vi "test_read-nmea-data2.vi"() -> ()   [LabVIEW 2019] (continued)
,12,307,21,1*5E\n\t\n15:09:51.45\tF9P\t$GPGSV,3,1,09,02,54,318,,04,19,044,,05,36,246,21,06,65,046,22,6*69\n\t\n15:09:51.47\tF9P\t$GPGSV,3,2,09,09,45,075,22,12,24,278,,17,34,153,,19,53,156,,6*63\n\t\n15:09:51.49\tF9P\t$GPGSV,3,3,09,25,12,307,,6*5A\n\t\n15:09:51.51\tF9P\t$GLGSV,2,1,08,69,13,031,,70,73,042,,71,50,204,27,72,03,209,,1*74\n\t\n15:09:51.53\tF9P\t$GLGSV,2,2,08,77,01,327,,84,21,121,08,85,70,063,24,86,35,329,,1*7B\n\t\n15:09:51.55\tF9P\t$GLGSV,2,1,08,69,13,031,,70,73,042,,71,50,204,21,72,03,209,,3*70\n\t\n15:09:51.57\tF9P\t$GLGSV,2,2,08,77,01,327,,84,21,121,12,85,70,063,18,86,35,329,,3*7D\n\t\n15:09:51.59\tF9P\t$GAGSV,2,1,08,02,09,298,,04,66,119,25,09,31,193,36,11,71,357,24,7*7E\n\t\n15:09:51.61\tF9P\t$GAGSV,2,2,08,12,40,102,17,19,27,045,10,25,09,249,,36,25,308,31,7*7E\n\t\n15:09:51.63\tF9P\t$GAGSV,2,1,08,02,09,298,,04,66,119,21,09,31,193,20,11,71,357,20,2*7C\n\t\n15:09:51.65\tF9P\t$GAGSV,2,2,08,12,40,102,,19,27,045,,25,09,249,,36,25,308,,2*7E\n\t\n15:09:51.67\tF9P\t$GBGSV,1,1,03,11,51,130,33,14,86,148,28,33,59,218,26,1*4C\n\t\n15:09:51.69\tF9P\t$GBGSV,1,1,04,08,,,22,11,51,130,25,14,86,148,21,33,59,218,,3*4B\n\t\n15:09:51.71\tF9P\t$GNGLL,3723.58734,N,12656.89105,E,060953.00,A,A*75\n\t\n15:09:51.73\tF9P\t\t\n15:09:51.75\tF9P\t\t\n15:09:51.77\tF9P\t\t\n15:09:51.79\tF9P\t\t\n15:09:51.81\tF9P\t\t\n15:09:51.83\tF9P\t\t\n15:09:51.85\tF9P\t\t\n15:09:51.87\tF9P\t\t\n15:09:51.89\tF9P\t\t\n15:09:51.91\tF9P\t\t\n15:09:51.93\tF9P\t\t\n15:09:51.95\tF9P\t\t\n15:09:51.97\tF9P\t\t\n15:09:51.99\tF9P\t\t\n15:09:52.01\tF9P\t\t\n15:09:52.03\tF9P\t\t\n15:09:52.05\tF9P\t\t\n15:09:52.07\tF9P\t\t\n15:09:52.09\tF9P\t\t\n15:09:52.11\tF9P\t\t\n15:09:52.13\tF9P\t\t\n15:09:52.15\tF9P\t\t\n15:09:52.17\tF9P\t\t\n15:09:52.19\tF9P\t\t\n15:09:52.21\tF9P\t\t\n15:09:52.23\tF9P\t\t\n15:09:52.25\tF9P\t$GNRMC,060954.00,A,3723.58684,N,12656.89052,E,0.440,,250720,,,A,V*1A\n\t\n15:09:52.27\tF9P\t$GNVTG,,T,,M,0.440,N,0.814,K,A*30\n\t\n15:09:52.29\tF9P\t$GNGGA,060954.00,3723.58684,N,12656.89052,E,1,12,0.74,39.4,M,18.5,M,,*7C\n\t\n15:09:52.31\tF9P\t$GNGSA,A,3,12,06,19,05,17,09,02,,,,,,1.38,0.74,1.16,1*0B\n\t\n15:09:52.33\tF9P\t$GNGSA,A,3,85,71,84,,,,,,,,,,1.38,0.74,1.16,2*0A\n\t\n15:09:52.35\tF9P\t$GNGSA,A,3,36,19,11,04,09,12,,,,,,,1.38,0.74,1.16,3*0F\n\t\n15:09:52.37\tF9P\t$GNGSA,A,3,14,11,33,,,,,,,,,,1.38,0.74,1.16,4*0E\n\t\n15:09:52.39\tF9P\t$GPGSV,3,1,09,02,54,318,32,04,19,044,,05,36,246,33,06,65,046,39,1*66\n\t\n15:09:52.41\tF9P\t$GPGSV,3,2,09,09,45,075,33,12,24,278,21,17,34,153,20,19,53,156,34,1*62\n\t\n15:09:52.43\tF9P\t$GPGSV,3,3,09,25,12,307,21,1*5E\n\t\n15:09:52.45\tF9P\t$GPGSV,3,1,09,02,54,318,,04,19,044,,05,36,246,21,06,65,046,29,6*62\n\t\n15:09:52.47\tF9P\t$GPGSV,3,2,09,09,45,075,22,12,24,278,,17,34,153,,19,53,156,,6*63\n\t\n15:09:52.49\tF9P\t$GPGSV,3,3,09,25,12,307,,6*5A\n\t\n15:09:52.51\tF9P\t$GLGSV,2,1,08,69,13,031,,70,73,042,,71,50,204,35,72,03,209,,1*77\n\t\n15:09:52.53\tF9P\t$GLGSV,2,2,08,77,01,327,,84,21,121,07,85,70,063,30,86,35,329,,1*71\n\t\n15:09:52.55\tF9P\t$GLGSV,2,1,08,69,13,031,,70,73,042,,71,50,204,21,72,03,209,,3*70\n\t\n15:09:52.57\tF9P\t$GLGSV,2,2,08,77,01,327,,84,21,121,12,85,70,063,27,86,35,329,,3*71\n\t\n15:09:52.59\tF9P\t$GAGSV,2,1,08,02,09,298,16,04,66,119,40,09,31,193,38,11,71,357,26,7*76\n\t\n15:09:52.61\tF9P\t$GAGSV,2,2,08,12,40,102,28,19,27,045,14,25,09,249,,36,25,308,32,7*75\n\t\n15:09:52.63\tF9P\t$GAGSV,2,1,08,02,09,298,,04,66,119,30,09,31,193,,11,71,357,23,2*7D\n\t\n15:09:52.65\tF9P\t$GAGSV,2,2,08,12,40,102,,19,27,045,,25,09,249,,36,25,308,,2*7E\n\t\n15:09:52.67\tF9P\t$GBGSV,1,1,03,11,50,131,45,14,86,148,37,33,59,218,33,1*47\n\t\n15:09:52.69\tF9P\t$GBGSV,1,1,04,08,,,29,11,50,131,25,14,86,148,,33,59,218,,3*43\n\t\n15:09:52.71\tF9P\t$GNGLL,3723.58684,N,12656.89052,E,060954.00,A,A*7B\n\t\n15:09:52.73\tF9P\t\t\n15:09:52.75\tF9P\t\t\n15:09:52.77\tF9P\t\t\n15:09:52.79\tF9P\t\t\n15:09:52.81\tF9P\t\t\n15:09:52.83\tF9P\t\t\n15:09:52.85\tF9P\t\t\n15:09:52.87\tF9P\t\t\n15:09:52.89\tF9P\t\t\n15:09:52.91\tF9P\t\t\n15:09:52.93\tF9P\t\t\n15:09:52.95\tF9P\t\t\n15:09:52.97\tF9P\t\t\n15:09:52.99\tF9P\t\t\n15:09:53.01\tF9P\t\t\n15:09:53.03\tF9P\t\t\n15:09:53.05\tF9P\t\t\n15:09:53.07\tF9P\t\t\n15:09:53.09\tF9P\t\t\n15:09:53.11\tF9P\t\t\n15:09:53.13\tF9P\t\t\n15:09:53.15\tF9P\t\t\n15:09:53.17\tF9P\t\t\n15:09:53.19\tF9P\t\t\n15:09:53.21\tF9P\t\t\n15:09:53.23\tF9P\t\t\n15:09:53.25\tF9P\t$GNRMC,060955.00,A,3723.58663,N,12656.88996,E,1.556,250.04,250720,,,A,V*08\n\t\n15:09:53.27\tF9P\t$GNVTG,250.04,T,,M,1.556,N,2.883,K,A*26\n\t\n15:09:53.29\tF9P\t$GNGGA,060955.00,3723.58663,N,12656.88996,E,1,12,0.78,38.7,M,18.5,M,,*7A\n\t\n15:09:53.31\tF9P\t$GNGSA,A,3,12,06,19,05,17,09,02,,,,,,1.55,0.78,1.34,1*0C\n\t\n15:09:53.33\tF9P\t$GNGSA,A,3,85,71,84,,,,,,,,,,1.55,0.78,1.34,2*0D\n\t\n15:09:53.35\tF9P\t$GNGSA,A,3,36,19,11,04,09,12,,,,,,,1.55,0.78,1.34,3*08\n\t\n15:09:53.37\tF9P\t$GNGSA,A,3,14,11,33,,,,,,,,,,1.55,0.78,1.34,4*09\n\t\n15:09:53.39\tF9P\t$GPGSV,3,1,09,02,54,318,32,04,19,044,20,05,36,246,36,06,65,046,38,1*60\n\t\n15:09:53.41\tF9P\t$GPGSV,3,2,09,09,45,075,34,12,24,278,21,17,34,153,23,19,53,156,28,1*6B\n\t\n15:09:53.43\tF9P\t$GPGSV,3,3,09,25,12,307,21,1*5E\n\t\n15:09:53.45\tF9P\t$GPGSV,3,1,09,02,54,318,,04,19,044,,05,36,246,21,06,65,046,22,6*69\n\t\n15:09:53.47\tF9P\t$GPGSV,3,2,09,09,45,075,23,12,24,278,,17,34,153,,19,53,156,,6*62\n\t\n15:09:53.49\tF9P\t$GPGSV,3,3,09,25,12,307,,6*5A\n\t\n15:09:53.51\tF9P\t$GLGSV,2,1,08,69,13,031,,70,73,042,,71,50,204,31,72,03,209,,1*73\n\t\n15:09:53.53\tF9P\t$GLGSV,2,2,08,77,01,327,,84,21,121,13,85,70,063,23,86,35,329,,1*76\n\t\n15:09:53.55\tF9P\t$GLGSV,2,1,08,69,13,031,,70,73,042,,71,50,204,29,72,03,209,,3*78\n\t\n15:09:53.57\tF9P\t$GLGSV,2,2,08,77,01,327,,84,21,121,16,85,70,063,21,86,35,329,,3*73\n\t\n15:09:53.59\tF9P\t$GAGSV,2,1,08,02,09,298,17,04,66,119,29,09,31,193,28,11,71,357,29,7*76\n\t\n15:09:53.61\tF9P\t$GAGSV,2,2,08,12,40,102,26,19,27,045,08,25,09,249,,36,25,308,27,7*72\n\t\n15:09:53.63\tF9P\t$GAGSV,2,1,08,02,09,298,,04,66,119,25,09,31,193,,11,71,357,22,2*78\n\t\n15:09:53.65\tF9P\t$GAGSV,2,2,08,12,40,102,,19,27,045,,25,09,249,,36,25,308,,2*7E\n\t\n15:09:53.67\tF9P\t$GBGSV,1,1,03,11,50,131,26,14,87,138,29,33,59,218,28,1*41\n\t\n15:09:53.69\tF9P\t$GBGSV,1,1,04,08,,,30,11,50,131,26,14,87,138,28,33,59,218,,3*44\n\t\n15:09:53.71\tF9P\t$GNGLL,3723.58663,N,12656.88996,E,060955.00,A,A*73\n\t\n15:09:53.73\tF9P\t\t\n15:09:53.75\tF9P\t\t\n15:09:53.77\tF9P\t\t\n15:09:53.79\tF9P\t\t\n15:09:53.81\tF9P\t\t\n15:09:53.83\tF9P\t\t\n15:09:53.85\tF9P\t\t\n15:09:53.87\tF9P\t\t\n15:09:53.89\tF9P\t\t\n15:09:53.91\tF9P\t\t\n15:09:53.93\tF9P\t\t\n15:09:53.95\tF9P\t\t\n15:09:53.97\tF9P\t\t\n15:09:53.99\tF9P\t\t\n15:09:54.01\tF9P\t\t\n15:09:54.03\tF9P\t\t\n15:09:54.05\tF9P\t\t\n15:09:54.07\tF9P\t\t\n15:09:54.09\tF9P\t\t\n15:09:54.11\tF9P\t\t\n15:09:54.13\tF9P\t\t\n15:09:54.15\tF9P\t\t\n15:09:54.17\tF9P\t\t\n15:09:54.19\tF9P\t\t\n15:09:54.21\tF9P\t\t\n15:09:54.23\tF9P\t\t\n15:09:54.25\tF9P\t$GNRMC,060956.00,A,3723.58624,N,12656.88943,E,1.511,240.62,250720,,,A,V*02\n\t\n15:09:54.27\tF9P\t$GNVTG,240.62,T,,M,1.511,N,2.799,K,A*20\n\t\n15:09:54.29\tF9P\t$GNGGA,060956.00,3723.58624,N,12656.88943,E,1,12,0.72,37.8,M,18.5,M,,*78\n\t\n15:09:54.31\tF9P\t$GNGSA,A,3,12,06,19,05,17,09,02,,,,,,1.36,0.72,1.16,1*03\n\t\n15:09:54.33\tF9P\t$GNGSA,A,3,85,71,84,,,,,,,,,,1.36,0.72,1.16,2*02\n\t\n15:09:54.35\tF9P\t$GNGSA,A,3,36,19,11,04,09,12,,,,,,,1.36,0.72,1.16,3*07\n\t\n15:09:54.37\tF9P\t$GNGSA,A,3,14,11,33,,,,,,,,,,1.36,0.72,1.16,4*06\n\t\n15:09:54.39\tF9P\t$GPGSV,3,1,09,02,54,318,28,04,19,044,20,05,36,246,29,06,65,046,38,1*65\n\t\n15:09:54.41\tF9P\t$GPGSV,3,2,09,09,45,075,31,12,24,278,22,17,34,153,22,19,53,156,26,1*62\n\t\n15:09:54.43\tF9P\t$GPGSV,3,3,09,25,12,307,22,1*5D\n\t\n15:09:54.45\tF9P\t$GPGSV,3,1,09,02,54,318,,04,19,044,,05,36,246,22,06,65,046,21,6*69\n\t\n15:09:54.47\tF9P\t$GPGSV,3,2,09,09,45,075,21,12,24,278,,17,34,153,,19,53,156,,6*60\n\t\n15:09:54.49\tF9P\t$GPGSV,3,3,09,25,12,307,,6*5A\n\t\n15:09:54.51\tF9P\t$GLGSV,2,1,08,69,13,031,,70,73,042,,71,50,204,26,72,03,209,,1*75\n\t\n15:09:54.53\tF9P\t$GLGSV,2,2,08,77,01,327,,84,21,121,10,85,70,063,29,86,35,329,,1*7F\n\t\n15:09:54.55\tF9P\t$GLGSV,2,1,08,69,13,031,,70,73,042,,71,50,204,22,72,03,209,,3*73\n\t\n15:09:54.57\tF9P\t$GLGSV,2,2,08,77,01,327,,84,21,121,18,85,70,063,21,86,35,329,,3*7D\n\t\n15:09:54.59\tF9P\t$GAGSV,2,1,08,02,09,298,16,04,66,119,26,09,31,193,27,11,71,357,26,7*78\n\t\n15:09:54.61\tF9P\t$GAGSV,2,2,08,12,40,102,22,19,27,045,13,25,09,249,,36,25,308,25,7*7E\n\t\n15:09:54.63\tF9P\t$GAGSV,2,1,08,02,09,298,,04,66,119,25,09,31,193,,11,71,357,20,2*7A\n\t\n15:09:54.65\tF9P\t$GAGSV,2,2,08,12,40,102,,19,27,045,,25,09,249,,36,25,308,,2*7E\n\t\n15:09:54.67\tF9P\t$GBGSV,2,1,05,11,50,131,27,12,,,21,14,87,138,22,15,,,22,1*77\n\t\n15:09:54.69\tF9P\t$GBGSV,2,2,05,33,59,218,31,1*46\n\t\n15:09:54.71\tF9P\t$GBGSV,1,1,03,11,50,131,25,14,87,138,27,33,59,218,,3*44\n\t\n15:09:54.73\tF9P\t$GNGLL,3723.58624,N,12656.88943,E,060956.00,A,A*7B\n\t\n15:09:54.75\tF9P\t\t\n15:09:54.77\tF9P\t\t\n15:09:54.79\tF9P\t\t\n15:09:54.81\tF9P\t\t\n15:09:54.83\tF9P\t\t\n15:09:54.85\tF9P\t\t\n15:09:54.87\tF9P\t\t\n15:09:54.89\tF9P\t\t\n15:09:54.91\tF9P\t\t\n15:09:54.93\tF9P\t\t\n15:09:54.95\tF9P\t\t\n15:09:54.97\tF9P\t\t\n15:09:54.99\tF9P\t\t\n15:09:55.01\tF9P\t\t\n15:09:55.03\tF9P\t\t\n15:09:55.05\tF9P\t\t\n15:09:55.07\tF9P\t\t\n15:09:55.09\tF9P\t\t\n15:09:55.11\tF9P\t\t\n15:09:55.13\tF9P\t\t\n15:09:55.15\tF9P\t\t\n15:09:55.17\tF9P\t\t\n15:09:55.19\tF9P\t\t\n15:09:55.21\tF9P\t\t\n15:09:55.23\tF9P\t\t\n15:09:55.25\tF9P\t$GNRMC,060957.00,A,3723.58600,N,12656.88891,E,1.206,,250720,,,A,V*16\n\t\n15:09:55.27\tF9P\t$GNVTG,,T,,M,1.206,N,2.234,K,A*3F\n\t\n15:09:55.29\tF9P\t$GNGGA,060957.00,3723.58600,N,12656.88891,E,1,12,0.72,37.6,M,18.5,M,,*7F\n\t\n15:09:55.31\tF9P\t$GNGSA,A,3,12,06,19,05,17,09,02,,,,,,1.36,0.72,1.16,1*03\n\t\n15:09:55.33\tF9P\t$GNGSA,A,3,85,71,84,,,,,,,,,,1.36,0.72,1.16,2*02\n\t\n15:09:55.35\tF9P\t$GNGSA,A,3,36,19,11,04,09,12,,,,,,,1.36,0.72,1.16,3*07\n\t\n15:09:55.37\tF9P\t$GNGSA,A,3,14,11,33,,,,,,,,,,1.36,0.72,1.16,4*06\n\t\n15:09:55.39\tF9P\t$GPGSV,3,1,09,02,54,318,27,04,19,044,19,05,36,246,29,06,65,046,32,1*6A\n\t\n15:09:55.41\tF9P\t$GPGSV,3,2,09,09,45,075,30,12,24,278,21,17,34,153,21,19,53,156,25,1*60\n\t\n15:09:55.43\tF9P\t$GPGSV,3,3,09,25,12,307,20,1*5F\n\t\n15:09:55.45\tF9P\t$GPGSV,3,1,09,02,54,318,,04,19,044,,05,36,246,21,06,65,046,21,6*6A\n\t\n15:09:55.47\tF9P\t$GPGSV,3,2,09,09,45,075,20,12,24,278,,17,34,153,,19,53,156,,6*61\n\t\n15:09:55.49\tF9P\t$GPGSV,3,3,09,25,12,307,,6*5A\n\t\n15:09:55.51\tF9P\t$GLGSV,2,1,08,69,13,031,,70,73,042,,71,50,204,27,72,03,209,,1*74\n\t\n15:09:55.53\tF9P\t$GLGSV,2,2,08,77,01,327,,84,21,121,07,85,70,063,29,86,35,329,,1*79\n\t\n15:09:55.55\tF9P\t$GLGSV,2,1,08,69,13,031,,70,73,042,,71,50,204,22,72,03,209,,3*73\n\t\n15:09:55.57\tF9P\t$GLGSV,2,2,08,77,01,327,,84,21,121,11,85,70,063,22,86,35,329,,3*77\n\t\n15:09:55.59\tF9P\t$GAGSV,2,1,08,02,09,298,15,04,66,119,25,09,31,193,28,11,71,357,25,7*74\n\t\n15:09:55.61\tF9P\t$GAGSV,2,2,08,12,40,102,18,19,27,045,18,25,09,249,,36,25,308,25,7*7C\n\t\n15:09:55.63\tF9P\t$GAGSV,2,1,08,02,09,298,,04,66,119,25,09,31,193,26,11,71,357,18,2*75\n\t\n15:09:55.65\tF9P\t$GAGSV,2,2,08,12,40,102,,19,27,045,,25,09,249,,36,25,308,,2*7E\n\t\n15:09:55.67\tF9P\t$GBGSV,1,1,03,11,50,131,26,14,87,138,22,33,60,219,27,1*4E\n\t\n15:09:55.69\tF9P\t$GBGSV,1,1,03,11,50,131,25,14,87,138,26,33,60,219,,3*4E\n\t\n15:09:55.71\tF9P\t$GNGLL,3723.58600,N,12656.88891,E,060957.00,A,A*72\n\t\n15:09:55.73\tF9P\t\t\n15:09:55.75\tF9P\t\t\n15:09:55.77\tF9P\t\t\n15:09:55.79\tF9P\t\t\n15:09:55.81\tF9P\t\t\n15:09:55.83\tF9P\t\t\n15:09:55.85\tF9P\t\t\n15:09:55.87\tF9P\t\t\n15:09:55.89\tF9P\t\t\n15:09:55.91\tF9P\t\t\n15:09:55.93\tF9P\t\t\n15:09:55.95\tF9P\t\t\n15:09:55.97\tF9P\t\t\n15:09:55.99\tF9P\t\t\n15:09:56.01\tF9P\t\t\n15:09:56.03\tF9P\t\t\n15:09:56.05\tF9P\t\t\n15:09:56.07\tF9P\t\t\n15:09:56.09\tF9P\t\t\n15:09:56.11\tF9P\t\t\n15:09:56.13\tF9P\t\t\n15:09:56.15\tF9P\t\t\n15:09:56.17\tF9P\t\t\n15:09:56.19\tF9P\t\t\n15:09:56.21\tF9P\t\t\n15:09:56.23\tF9P\t\t\n15:09:56.25\tF9P\t$GNRMC,060958.00,A,3723.58560,N,12656.88866,E,1.310,,250720,,,A,V*12\n\t\n15:09:56.27\tF9P\t$GNVTG,,T,,M,1.310,N,2.427,K,A*3D\n\t\n15:09:56.29\tF9P\t$GNGGA,060958.00,3723.58560,N,12656.88866,E,1,12,0.68,37.8,M,18.5,M,,*78\n\t\n15:09:56.31\tF9P\t$GNGSA,A,3,12,06,19,05,17,09,02,,,,,,1.28,0.68,1.09,1*09\n\t\n15:09:56.33\tF9P\t$GNGSA,A,3,85,71,84,,,,,,,,,,1.28,0.68,1.09,2*08\n\t\n15:09:56.35\tF9P\t$GNGSA,A,3,36,19,11,04,09,12,,,,,,,1.28,0.68,1.09,3*0D\n\t\n15:09:56.37\tF9P\t$GNGSA,A,3,14,11,33,,,,,,,,,,1.28,0.68,1.09,4*0C\n\t\n15:09:56.39\tF9P\t$GPGSV,3,1,09,02,54,318,26,04,19,044,16,05,36,246,28,06,65,046,32,1*65\n\t\n15:09:56.41\tF9P\t$GPGSV,3,2,09,09,45,075,30,12,24,278,20,17,34,153,20,19,53,156,24,1*61\n\t\n15:09:56.43\tF9P\t$GPGSV,3,3,09,25,12,307,19,1*55\n\t\n15:09:56.45\tF9P\t$GPGSV,3,1,09,02,54,318,,04,19,044,,05,36,246,21,06,65,046,22,6*69\n\t\n15:09:56.47\tF9P\t$GPGSV,3,2,09,09,45,075,19,12,24,278,,17,34,153,,19,53,156,,6*6B\n\t\n15:09:56.49\tF9P\t$GPGSV,3,3,09,25,12,307,,6*5A\n\t\n15:09:56.51\tF9P\t$GLGSV,2,1,08,69,13,031,,70,73,042,,71,50,204,25,72,03,209,,1*76\n\t\n15:09:56.53\tF9P\t$GLGSV,2,2,08,77,01,327,,84,21,121,07,85,70,063,23,86,35,329,,1*73\n\t\n15:09:56.55\tF9P\t$GLGSV,2,1,08,69,13,031,,70,73,042,,71,50,204,22,72,03,209,,3*73\n\t\n15:09:56.57\tF9P\t$GLGSV,2,2,08,77,01,327,,84,21,121,15,85,70,063,22,86,35,329,,3*73\n\t\n15:09:56.59\tF9P\t$GAGSV,2,1,08,02,09,298,13,04,66,119,23,09,31,193,25,11,71,357,24,7*78\n\t\n15:09:56.61\tF9P\t$GAGSV,2,2,08,12,40,102,19,19,27,045,14,25,09,249,,36,25,308,23,7*77\n\t\n15:09:56.63\tF9P\t$GAGSV,2,1,08,02,09,298,,04,66,119,24,09,31,193,22,11,71,357,20,2*7B\n\t\n15:09:56.65\tF9P\t$GAGSV,2,2,08,12,40,102,,19,27,045,,25,09,249,,36,25,308,,2*7E\n\t\n15:09:56.67\tF9P\t$GBGSV,1,1,03,11,50,131,25,14,87,138,23,33,60,219,27,1*4C\n\t\n15:09:56.69\tF9P\t$GBGSV,1,1,03,11,50,131,25,14,87,138,25,33,60,219,,3*4D\n\t\n15:09:56.71\tF9P\t$GNGLL,3723.58560,N,12656.88866,E,060958.00,A,A*70\n\t\n15:09:56.73\tF9P\t\t\n15:09:56.75\tF9P\t\t\n15:09:56.77\tF9P\t\t\n15:09:56.79\tF9P\t\t\n15:09:56.81\tF9P\t\t\n15:09:56.83\tF9P\t\t\n15:09:56.85\tF9P\t\t\n15:09:56.87\tF9P\t\t\n15:09:56.89\tF9P\t\t\n15:09:56.91\tF9P\t\t\n15:09:56.93\tF9P\t\t\n15:09:56.95\tF9P\t\t\n15:09:56.97\tF9P\t\t\n15:09:56.99\tF9P\t\t\n15:09:57.01\tF9P\t\t\n15:09:57.03\tF9P\t\t\n15:09:57.05\tF9P\t\t\n15:09:57.07\tF9P\t\t\n15:09:57.09\tF9P\t\t\n15:09:57.11\tF9P\t\t\n15:09:57.13\tF9P\t\t\n15:09:57.15\tF9P\t\t\n15:09:57.17\tF9P\t\t\n15:09:57.19\tF9P\t\t\n15:09:57.21\tF9P\t\t\n15:09:57.23\tF9P\t\t\n15:09:57.25\tF9P\t$GNRMC,060959.00,A,3723.58525,N,12656.88852,E,0.881,,250720,,,A,V*17\n\t\n15:09:57.27\tF9P\t$GNVTG,,T,,M,0.881,N,1.631,K,A*39\n\t\n15:09:57.29\tF9P\t$GNGGA,060959.00,3723.58525,N,12656.88852,E,1,12,0.67,37.6,M,18.5,M,,*7E\n\t\n15:09:57.31\tF9P\t$GNGSA,A,3,12,06,19,05,17,09,04,02,,,,,1.29,0.67,1.10,1*0B\n\t\n15:09:57.33\tF9P\t$GNGSA,A,3,85,71,,,,,,,,,,,1.29,0.67,1.10,2*02\n\t\n15:09:57.35\tF9P\t$GNGSA,A,3,36,19,11,04,09,12,,,,,,,1.29,0.67,1.10,3*0B\n\t\n15:09:57.37\tF9P\t$GNGSA,A,3,14,11,33,,,,,,,,,,1.29,0.67,1.10,4*0A\n\t\n15:09:57.39\tF9P\t$GPGSV,3,1,09,02,54,318,24,04,19,044,15,05,36,246,20,06,65,046,31,1*6F\n\t\n15:09:57.41\tF9P\t$GPGSV,3,2,09,09,45,075,25,12,24,278,19,17,34,153,18,19,53,156,25,1*65\n\t\n15:09:57.43\tF9P\t$GPGSV,3,3,09,25,12,307,18,1*54\n\t\n15:09:57.45\tF9P\t$GPGSV,3,1,09,02,54,318,,04,19,044,,05,36,246,19,06,65,046,22,6*62\n\t\n15:09:57.47\tF9P\t$GPGSV,3,2,09,09,45,075,18,12,24,278,,17,34,153,,19,53,156,,6*6A\n\t\n15:09:57.49\tF9P\t$GPGSV,3,3,09,25,12,307,,6*5A\n\t\n15:09:57.51\tF9P\t$GLGSV,2,1,08,69,13,031,,70,73,042,,71,50,204,24,72,03,209,,1*77\n\t\n15:09:57.53\tF9P\t$GLGSV,2,2,08,77,01,327,,84,21,121,06,85,70,063,23,86,35,329,,1*72\n\t\n15:09:57.55\tF9P\t$GLGSV,2,1,08,69,13,031,,70,73,042,,71,50,204,22,72,03,209,,3*73\n\t\n15:09:57.57\tF9P\t$GLGSV,2,2,08,77,01,327,,84,21,121,07,85,70,063,22,86,35,329,,3*70\n\t\n15:09:57.59\tF9P\t$GAGSV,2,1,08,02,09,298,11,04,66,119,25,09,31,193,24,11,71,357,23,7*7A\n\t\n15:09:57.61\tF9P\t$GAGSV,2,2,08,12,40,102,20,19,27,045,19,25,09,249,,36,25,308,23,7*70\n\t\n15:09:57.63\tF9P\t$GAGSV,2,1,08,02,09,298,,04,66,119,22,09,31,193,20,11,71,357,19,2*75\n\t\n15:09:57.65\tF9P\t$GAGSV,2,2,08,12,40,102,,19,27,045,,25,09,249,,36,25,308,,2*7E\n\t\n15:09:57.67\tF9P\t$GBGSV,1,1,03,11,50,131,23,14,87,138,22,33,60,219,28,1*44\n\t\n15:09:57.69\tF9P\t$GBGSV,1,1,03,11,50,131,23,14,87,138,23,33,60,219,,3*4D\n\t\n15:09:57.71\tF9P\t$GNGLL,3723.58525,N,12656.88852,E,060959.00,A,A*77\n\t\n15:09:57.73\tF9P\t\t\n15:09:57.75\tF9P\t\t\n15:09:57.77\tF9P\t\t\n15:09:57.79\tF9P\t\t\n15:09:57.81\tF9P\t\t\n15:09:57.83\tF9P\t\t\n15:09:57.85\tF9P\t\t\n15:09:57.87\tF9P\t\t\n15:09:57.89\tF9P\t\t\n15:09:57.91\tF9P\t\t\n15:09:57.93\tF9P\t\t\n15:09:57.95\tF9P\t\t\n15:09:57.97\tF9P\t\t\n15:09:57.99\tF9P\t\t\n15:09:58.01\tF9P\t\t\n15:09:58.03\tF9P\t\t\n15:09:58.05\tF9P\t\t\n15:09:58.07\tF9P\t\t\n15:09:58.09\tF9P\t\t\n15:09:58.11\tF9P\t\t\n15:09:58.13\tF9P\t\t\n15:09:58.15\tF9P\t\t\n15:09:58.17\tF9P\t\t\n15:09:58.19\tF9P\t\t\n15:09:58.21\tF9P\t\t\n15:09:58.23\tF9P\t\t\n15:09:58.25\tF9P\t$GNRMC,061000.00,A,3723.58497,N,12656.88781,E,2.064,,250720,,,A,V*1B\n\t\n15:09:58.27\tF9P\t$GNVTG,,T,,M,2.064,N,3.822,K,A*36\n\t\n15:09:58.29\tF9P\t$GNGGA,061000.00,3723.58497,N,12656.88781,E,1,12,0.64,37.9,M,18.5,M,,*7F\n\t\n15:09:58.31\tF9P\t$GNGSA,A,3,12,06,19,05,17,09,04,02,,,,,1.19,0.64,1.00,1*0A\n\t\n15:09:58.33\tF9P\t$GNGSA,A,3,85,71,84,,,,,,,,,,1.19,0.64,1.00,2*0F\n\t\n15:09:58.35\tF9P\t$GNGSA,A,3,36,19,11,04,09,12,,,,,,,1.19,0.64,1.00,3*0A\n\t\n15:09:58.37\tF9P\t$GNGSA,A,3,14,11,33,,,,,,,,,,1.19,0.64,1.00,4*0B\n\t\n15:09:58.39\tF9P\t$GPGSV,3,1,09,02,54,318,24,04,19,044,16,05,36,246,22,06,65,046,32,1*6D\n\t\n15:09:58.41\tF9P\t$GPGSV,3,2,09,09,45,075,27,12,24,278,19,17,34,153,20,19,53,156,25,1*6C\n\t\n15:09:58.43\tF9P\t$GPGSV,3,3,09,25,12,307,17,1*5B\n\t\n15:09:58.45\tF9P\t$GPGSV,3,1,09,02,54,318,,04,19,044,,05,36,246,16,06,65,046,22,6*6D\n\t\n15:09:58.47\tF9P\t$GPGSV,3,2,09,09,45,075,18,12,24,278,,17,34,153,,19,53,156,,6*6A\n\t\n15:09:58.49\tF9P\t$GPGSV,3,3,09,25,12,307,,6*5A\n\t\n15:09:58.51\tF9P\t$GLGSV,2,1,08,69,13,031,,70,73,042,,71,50,204,21,72,03,209,,1*72\n\t\n15:09:58.53\tF9P\t$GLGSV,2,2,08,77,01,327,,84,21,121,08,85,70,063,24,86,35,329,,1*7B\n\t\n15:09:58.55\tF9P\t$GLGSV,2,1,08,69,13,031,,70,73,042,,71,50,204,22,72,03,209,,3*73\n\t\n15:09:58.57\tF9P\t$GLGSV,2,2,08,77,01,327,,84,21,121,10,85,70,063,22,86,35,329,,3*76\n\t\n15:09:58.59\tF9P\t$GAGSV,2,1,08,02,09,298,13,04,66,119,25,09,31,193,20,11,71,357,22,7*7D\n\t\n15:09:58.61\tF9P\t$GAGSV,2,2,08,12,40,102,19,19,27,045,14,25,09,249,,36,25,308,20,7*74\n\t\n15:09:58.63\tF9P\t$GAGSV,2,1,08,02,09,298,,04,66,119,22,09,31,193,17,11,71,357,19,2*71\n\t\n15:09:58.65\tF9P\t$GAGSV,2,2,08,12,40,102,,19,27,045,,25,09,249,,36,25,308,,2*7E\n\t\n15:09:58.67\tF9P\t$GBGSV,1,1,03,11,50,131,21,14,87,138,20,33,60,219,25,1*49\n\t\n15:09:58.69\tF9P\t$GBGSV,1,1,03,11,50,131,22,14,87,138,23,33,60,219,,3*4C\n\t\n15:09:58.71\tF9P\t$GNGLL,3723.58497,N,12656.88781,E,061000.00,A,A*7A\n\t\n15:09:58.73\tF9P\t\t\n15:09:58.75\tF9P\t\t\n15:09:58.77\tF9P\t\t\n15:09:58.79\tF9P\t\t\n15:09:58.81\tF9P\t\t\n15:09:58.83\tF9P\t\t\n15:09:58.85\tF9P\t\t\n15:09:58.87\tF9P\t\t\n15:09:58.89\tF9P\t\t\n15:09:58.91\tF9P\t\t\n15:09:58.93\tF9P\t\t\n15:09:58.95\tF9P\t\t\n15:09:58.97\tF9P\t\t\n15:09:58.99\tF9P\t\t\n15:09:59.01\tF9P\t\t\n15:09:59.03\tF9P\t\t\n15:09:59.05\tF9P\t\t\n15:09:59.07\tF9P\t\t\n15:09:59.09\tF9P\t\t\n15:09:59.11\tF9P\t\t\n15:09:59.13\tF9P\t\t\n15:09:59.15\tF9P\t\t\n15:09:59.17\tF9P\t\t\n15:09:59.19\tF9P\t\t\n15:09:59.21\tF9P\t\t\n15:09:59.23\tF9P\t\t\n15:09:59.25\tF9P\t$GNRMC,061001.00,A,3723.58468,N,12656.88727,E,1.242,,250720,,,A,V*13\n\t\n15:09:59.27\tF9P\t$GNVTG,,T,,M,1.242,N,2.301,K,A*38\n\t\n15:09:59.29\tF9P\t$GNGGA,061001.00,3723.58468,N,12656.88727,E,1,12,0.68,38.6,M,18.5,M,,*7E\n\t\n15:09:59.31\tF9P\t$GNGSA,A,3,12,06,19,05,17,09,04,02,,,,,1.28,0.68,1.09,1*0D\n
